vi "Passive Force Clamp-final-v1.vi"(4 "file name add to the end (height)":string="h300", 5 "feedback?":bool, 6 "X=T,Y=F":bool=TRUE, 7 "save?":bool, 8 "Intensity Control, 0~-7000 (mV)":dbl=-1200.0 format="%_8g", 9 "moving step size (um)":dbl=0.05, 10 "upper set value":dbl=0.34, 11 "range (um)":dbl=2.0 format="%.3f") -> ()   [LabVIEW 2014]
uses:
  <vilib>/Analysis/baseanly.llb/Mean (DBL).vi
  Main-Stage-PI/(Global) Current handle and LaserPower_YCC.vi
  <vilib>/Analysis/NI_AALBase.lvlib
panel:
  in  "Custom choose?":bool
  out "Jump to middle (um)":dbl
  out "Max QPD-Stage Pos (um)":dbl
  in  "lower set value":dbl=0.26
  out "target QPD (V)":dbl
  in  "Avg. time delay (ms)":dbl=20.0
  out "True Target position":dbl
  in  "averged delay":dbl
  out "Record scan rate  (um/s)":dbl=2.0
  out "Laser Lock?":bool
  out "Center QPD yc (V)":dbl format="%0.2f"
  out "Sampling rate after filtering (Hz)":dbl
  in  "Who's Data":enum16{"YCC", "PYW", "LCH", "YYH"}(ring)
  in  "left rank":i32=160
  out "Stage-QPD data":dbl[][](array[numeric])
  out "Now position (um)":dbl
  in  "Avg points":i32=320
  out "True rate?":bool
  out "Real initial position (um)":dbl format="%0.5f"
  out "Axis":i32
  in  "toward+ ?\nT=+, F=-":bool
  out "target position (um)":dbl
  in  "stop":bool
  in  "Tab Control":enum32{"Stage movment", "Raw Data", "All Data"}(tab)
  out "XY Graph":T1(graph)
  in  "Set Target position?":bool
  out "Z-QPD":dbl(graph)
  out "Waveform Chart":dbl[](graph)
  out "XY Graph 2":cluster{dbl[], "Filtered X":dbl[]}[](graph)
  in  "Sampling rate":dbl=32000.0
  # "20R-- 300mV"
  # "peak~350 nm\nfrom r = 400 to 500 nm"
  # "jump to r=450 nm"
  # "2.9um for had acted"
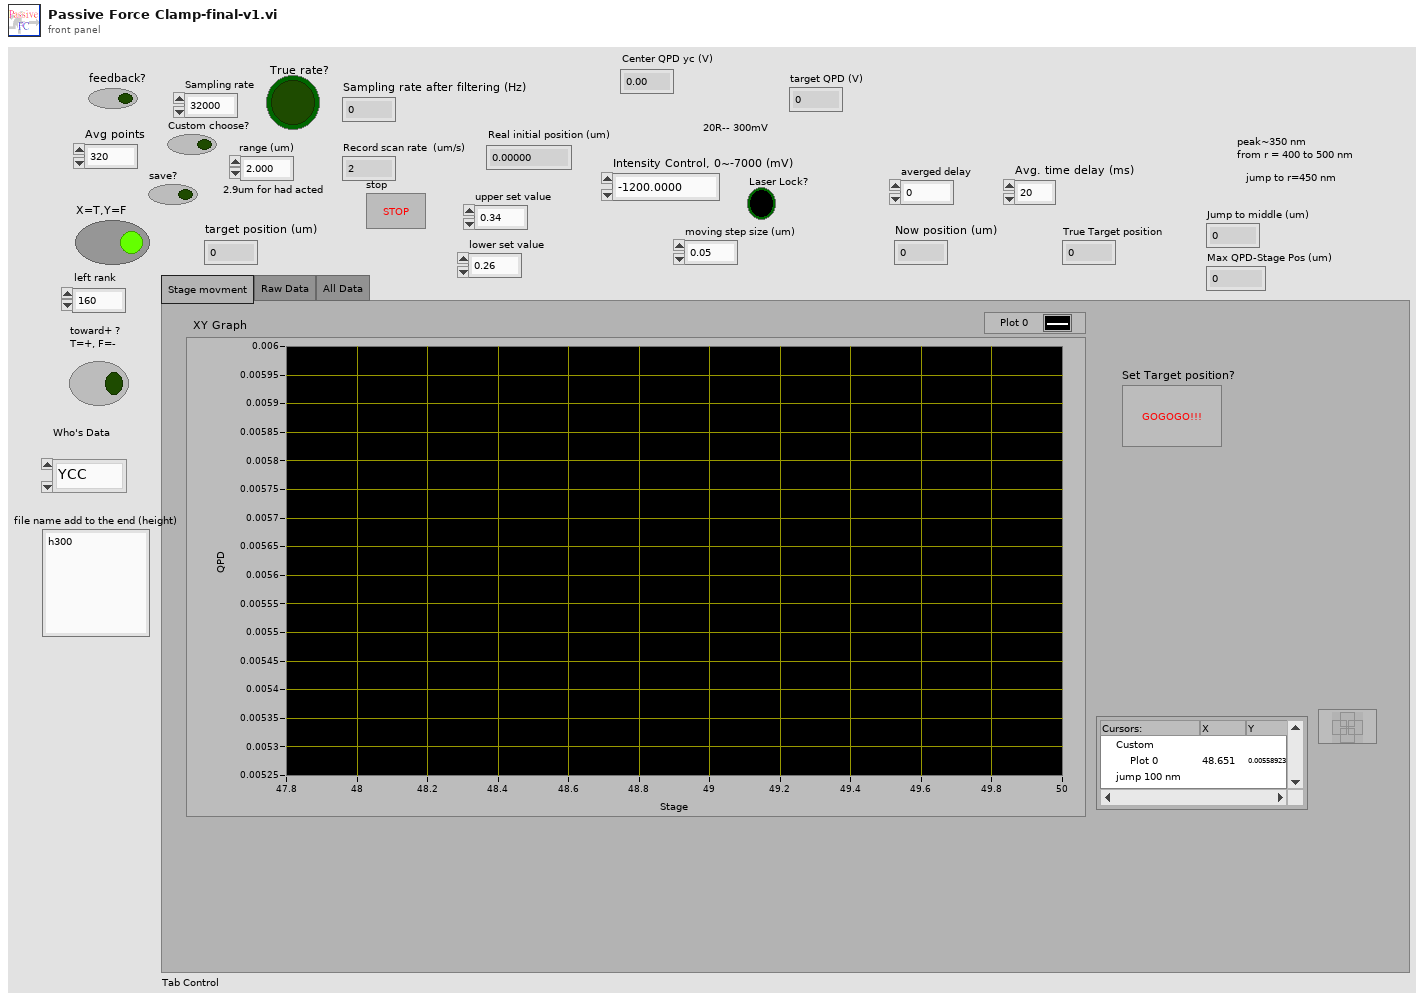
[diagram p1: front panel]
types:
  T1 = cluster{"Filtered Stage Array":dbl[], "Filtered QPD data":dbl[]}
  T2 = enum16{"Fixed-window avg", "Moving-window avg", "F+S-window avg", "S-G filter", "Fixed-window Median", "Moving-window Median "}
  T3 = cluster{"Correct Unfolded Stage Array (um)":dbl[], "Filtered QPD Array":dbl[]}
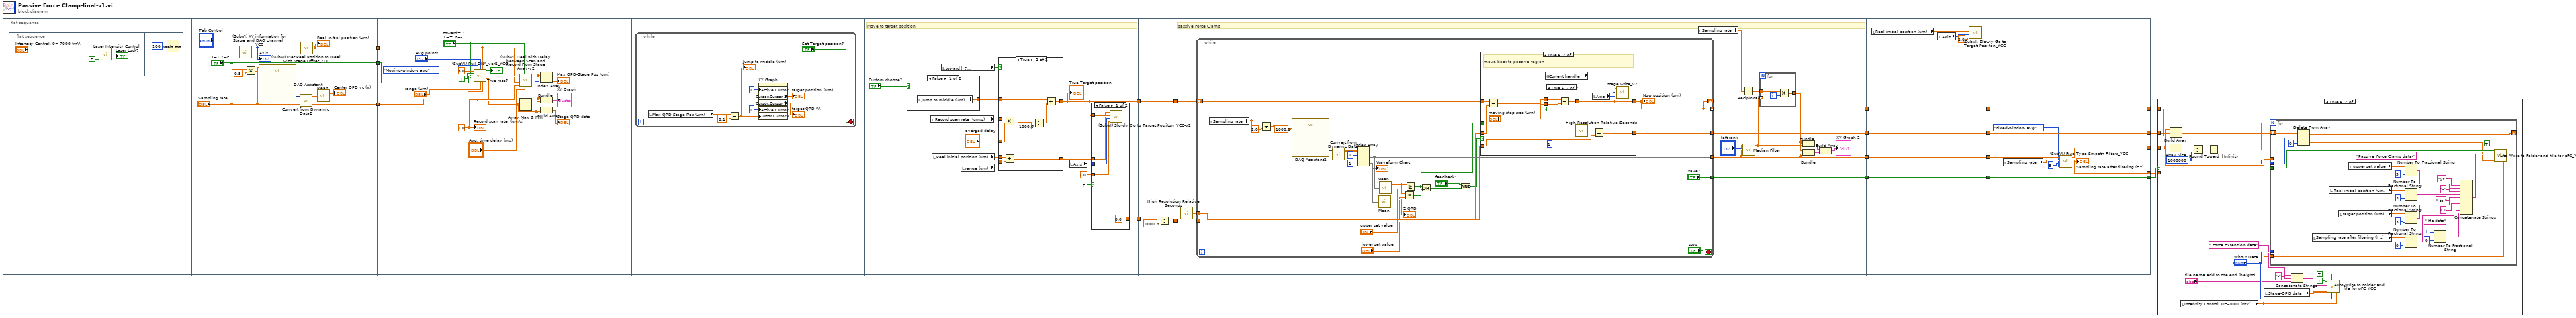
[diagram p0: block diagram]
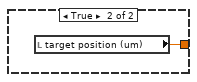
[diagram p3: hidden frame]
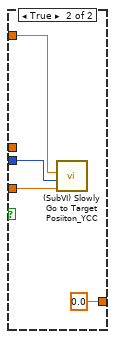
[diagram p4: hidden frame]
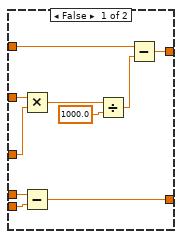
[diagram p5: hidden frame]
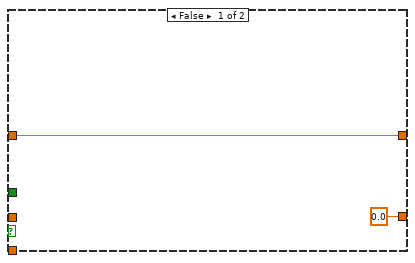
[diagram p6: hidden frame]
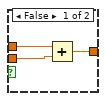
[diagram p7: hidden frame]
diagram:
  n1 = flat-sequence {
    tunnel: [w32] -> w17
    tunnel: ["X=T,Y=F"] -> w16
    tunnel: ["Sampling rate"] -> w5
    tunnel: w17 -> [w40]
    tunnel: w16 -> [w45]
    tunnel: w5 -> [w44]
    tunnel: [w68] -> w15
    tunnel: [w73] -> w4
    tunnel: w15 -> [w108]
    tunnel: [w108] -> w14
    tunnel: [w106] -> w13
    tunnel: w4 -> [w105]
    tunnel: w14 -> [w120]
    tunnel: w13 -> [w119]
    tunnel: [w113] -> w11
    tunnel: [w122] -> w9
    tunnel: [w121] -> w7
    tunnel: [w109] -> w2
    tunnel: w11 -> [w178]
    tunnel: [w178] -> w10
    tunnel: w9 -> [w177]
    tunnel: [w177] -> w8
    tunnel: w7 -> [w176]
    tunnel: [w176] -> w6
    tunnel: [w172] -> w3
    tunnel: w2 -> [w172]
    tunnel: [w186] -> w18
    tunnel: [w187] -> w19
    tunnel: [w181] -> w20
    tunnel: w10 -> [w185]
    tunnel: w8 -> [w187]
    tunnel: w6 -> [w186]
    tunnel: [w182] -> w12
    tunnel: w3 -> [w179]
    tunnel: [w179] -> w1
    frame #0 {
      n2 = flat-sequence {
        frame #0 {
          n3 = call "Laser Intensity Control.vi"("Close?"=FALSE, "Intensity Control, 0~-7000 (mV)"="Intensity Control, 0~-7000 (mV)") -> ("Laser Lock?"=→"Laser Lock?":bool)  [unwired: 5 in]
        }
        frame #1 {
          n4 = Wait (ms)(milliseconds to wait=u32 100) -> ()  [unwired: 1 out]
        }
      }
    }
    frame #1 {
      n5 = call "(SubVI) XY information for Stage and DAQ channel_YCC.vi"("T=X\nF=Y"="X=T,Y=F") -> ("Axis"=w33:i32)  [unwired: 3 in, 1 out]
      "Axis" <- w33
      n6 = Multiply(x="Sampling rate", y=0.5) -> (x*y=w28:dbl)
      n7 = call "DAQ Assistant"("rate"="Sampling rate", "number of samples"=w28) -> ("data"=w27:dynamicdata)  [unwired: 15 in, 2 out]
      n8 = call "Convert from Dynamic Data2"("Dynamic Data Type"=w27) -> ("Array"=w26:dbl[])  [unwired: 3 in]
      n9 = call "(SubVI) Get Real Position to Deal with Stage Offset_YCC.vi"("Axis"=w33) -> ("Real Current Commanded position (um)"=w32:dbl)  [unwired: 3 in, 1 out]
      "Real initial position (um)" <- w32
      n10 = call-poly <vilib>:"Mean.vi"("X"=w26) -> ("mean"=→"Center QPD yc (V)":dbl)  [unwired: 1 out]
    }
    frame #2 {
      w39 = 1.0 ("Record scan rate  (um/s)")
      n11 = call "(SubVI) Pull DNA_ver2_YCC.vi"("waiting time per point (ms)\nrange from 5ms to 0.167 ms"=5.0 ("waiting time per point (ms)\nrange from 5ms to 0.167 ms"), "Filter type"=T2."Moving-window avg", "Avg points"="Avg points", "Real initial position (um)"=w40, "Record?"=TRUE, "T=X\nF=Y"=w45, "Toward  ?\nT=+, F=-"="toward+ ?\nT=+, F=-", "Record scan rate  (um/s)"=w39, "range  (um)"="range (um)", "Sampling rate"=w44) -> ("True rate?"=→"True rate?":bool, "Filtered Stage Array"=w42:dbl[], "Filtered QPD Array"=w37:dbl[])  [unwired: 2 in, 1 out]
      n12 = call "(SubVI) Deal with Delay between Scan and Record From Stage Array-v2.vi"("Avg. time delay (ms)"="Avg. time delay (ms)", "Toward first ?\nT=+, F=-"="toward+ ?\nT=+, F=-", "Record scan rate  (um/s)"=w39, "Real initial position (um)"=w40, "Unfolded Stage Array (um)"=w42) -> ("Correct Unfolded Stage Array (um)"=w36:dbl[])  [unwired: 2 in, 2 out]
      n13 = Array Max & Min(array=w37) -> (max index (indices)=w35:i32)  [unwired: 3 out]
      n14 = Index Array(array=w36, index=w35) -> (element=→"Max QPD-Stage Pos (um)":dbl)
      n15 = Bundle("Correct Unfolded Stage Array (um)"=w36, "Filtered QPD Array"=w37) -> (→"XY Graph":T3)  [unwired: 1 in]
      n16 = Build Array(w36, w37) -> (→"Stage-QPD data":dbl[][])
      "Record scan rate  (um/s)" <- w39
    }
    frame #3 {
      n17 = while {
        stop <- "Set Target position?" stop-if-true
        n18 = local read "Max QPD-Stage Pos (um)"() -> (w55:dbl)
        n19 = Subtract(x=w55, y=0.1) -> (x-y=w53:dbl)
        "Jump to middle (um)" <- w53
        n20 = property on="XY Graph" class="XYGraph (strict)"("Active Cursor"=u32 0, "Active Cursor"=u32 1, "Cursor.Cursor X"=w53) -> ("Cursor.Cursor X"=→"target position (um)":dbl, "Cursor.Cursor Y"=→"target QPD (V)":dbl)  [unwired: 2 in, 2 out]
      }
    }
    frame #4 {
      # "Move to target position"
      n21 = case shown="False" "Custom choose?" {
        tunnel: [w74 w75] -> w72
        frame False {
          n22 = local read "Jump to middle (um)"() -> (w74:dbl)
        }
        frame True {
          n23 = local read "target position (um)"() -> (w75:dbl)
        }
      }
      n24 = local read "Record scan rate  (um/s)"() -> (w69:dbl)
      n25 = local read "Real initial position (um)"() -> (w64:dbl)
      n26 = local read "toward+ ?\nT=+, F=-"() -> (w71:bool)
      n27 = local read "range (um)"() -> (w63:dbl)
      n28 = case shown="True" w71 {
        tunnel: w72 -> [w94 w100]
        tunnel: [w90 w98] -> w68
        tunnel: "averged delay" -> [w89 w101]
        tunnel: w69 -> [w88 w102]
        tunnel: w64 -> [w87 w97]
        tunnel: w63 -> [w86 w96]
        tunnel: [w85 w95] -> w62
        frame False {
          n29 = Multiply(x=w88, y=w89) -> (x*y=w93:dbl)
          n30 = Subtract(x=w87, y=w86) -> (x-y=w85:dbl)
          n31 = Divide(x=w93, y=1000.0) -> (x/y=w91:dbl)
          n32 = Subtract(x=w94, y=w91) -> (x-y=w90:dbl)
        }
        frame True {
          n33 = Multiply(x=w102, y=w101) -> (x*y=w104:dbl)
          n34 = Add(x=w97, y=w96) -> (x+y=w95:dbl)
          n35 = Divide(x=w104, y=1000.0) -> (x/y=w99:dbl)
          n36 = Add(x=w100, y=w99) -> (x+y=w98:dbl)
        }
      }
      "True Target position" <- w68
      n37 = local read "Axis"() -> (w66:i32)
      n38 = case shown="False" FALSE {
        tunnel: [0.0 ("Expect - Real move (nm)\nStage Offset\n+=more move\n-=less move") 0.0 ("Expect - Real move (nm)\nStage Offset\n+=more move\n-=less move")] -> w73
        tunnel: w68 -> [w79 w84]
        tunnel: w66 -> [w78 w82]
        tunnel: 1.0 ("scan rate  (um/s)") -> [w77 w81]
        tunnel: w62 -> [w76 _]
        frame False {
          n39 = call "(SubVI) Slowly Go to Target Posiiton_YCC-v2.vi"("scan rate  (um/s)"=w77, "axis"=w78, "Target position (um)"=w79, "Now position (um)"=w76) -> ()  [unwired: 2 in, 2 out]
        }
        frame True {
          n40 = call "(SubVI) Slowly Go to Target Posiiton_YCC.vi"("scan rate  (um/s)"=w81, "axis"=w82, "Target position (um)"=w84) -> ()  [unwired: 1 in, 4 out]
        }
      }
    }
    frame #5 {
      n41 = Divide(x=w105, y=1000.0) -> (x/y=w106:dbl)
    }
    frame #6 {
      # "passive Force Clamp"
      n42 = call <vilib>:"High Resolution Relative Seconds.vi"() -> ("relative seconds"=w123:dbl)
      n43 = while {
        tunnel: w123 -> [w149]
        tunnel: [w148] -> w122 mode=indexing
        tunnel: [w135] -> w113 mode=concatenating
        tunnel: ["save?"] -> w121
        shift-right: [w127] -> _
        shift-left: w120 -> [w139]
        tunnel: w119 -> [w140]
        tunnel: [w127] -> w109 mode=indexing
        stop <- "stop" stop-if-true
        n44 = local read "Sampling rate"() -> (w143:dbl)
        n45 = Divide(x=w143, y=2.0) -> (x/y=w141:dbl)
        n46 = call "DAQ Assistant2"("rate"=w143, "number of samples"=w141, "timeout (s)"=1000.0) -> ("data"=w146:dynamicdata)  [unwired: 13 in, 3 out]
        n47 = call "Convert from Dynamic Data"("Dynamic Data Type"=w146) -> ("Array"=w138:dbl[][])  [unwired: 3 in]
        n48 = Index Array(array=w138, index (row) #1=0 ("index (row)"), index (row) #2=1 ("index (row)")) -> (element #1=w135:dbl[], element #2=w134:dbl[])  [unwired: 2 in]
        "Waveform Chart" <- w135
        n49 = call-poly <vilib>:"Mean.vi"("X"=w134) -> ("mean"=→"Z-QPD":dbl)  [unwired: 1 out]
        n50 = call-poly <vilib>:"Mean.vi"("X"=w135) -> ("mean"=w151:dbl)  [unwired: 1 out]
        n51 = Less Or Equal?(x=w151, y="lower set value") -> (x <= y?=w130:bool)
        n52 = Greater Or Equal?(x=w151, y="upper set value") -> (x >= y?=w128:bool)
        n53 = Or(x=w128, y=w130) -> (x .or. y?=w129:bool)
        n54 = And(x="feedback?", y=w129) -> (x .and. y?=w131:bool)
        n55 = case shown="True" w131 {
          tunnel: w149 -> [_ w164]
          tunnel: [0.0 w162] -> w148
          tunnel: [w153 w161] -> w127
          tunnel: w140 -> [_ w159]
          tunnel: w139 -> [w153 w156]
          tunnel: w128 -> [_ w155]
          frame False {
          }
          frame True {
            (unwired) 1 ("read #")
            # "move back to passive region"
            n56 = Subtract(x=w156, y=w159) -> (x-y=w158:dbl)
            n57 = case shown="True" w155 {
              tunnel: "moving step size (um)" -> [w166 w171]
              tunnel: [w168 w170] -> w161
              tunnel: w158 -> [w167 w169]
              frame False {
                n58 = Add(x=w167, y=w166) -> (x+y=w168:dbl)
              }
              frame True {
                n59 = Subtract(x=w169, y=w171) -> (x-y=w170:dbl)
              }
            }
            n60 = global read "(Global) Current handle and LaserPower_YCC.vi" "Current handle"() -> (w157:i32)
            n61 = call <vilib>:"High Resolution Relative Seconds.vi"() -> ("relative seconds"=w163:dbl)
            n62 = local read "Axis"() -> (w160:i32)
            n63 = Subtract(x=w163, y=w164) -> (x-y=w162:dbl)
            n64 = call "stage write_v2.vi"("axis"=w160, "Incoming Handle"=w157, "position"=w161) -> ()  [unwired: 2 in, 1 out]
          }
        }
        "Now position (um)" <- w127
      }
      n65 = local read "Sampling rate"() -> (w117:dbl)
      n66 = Reciprocal(x=w117) -> (1/x=w116:dbl)
      n67 = call <vilib>:"Median Filter.vi"("left rank"="left rank", "X"=w113) -> ("Filtered X"=w115:dbl[])  [unwired: 8 in, 1 out]
      n68 = for {
        tunnel: w115 -> [_] mode=indexing
        tunnel: w116 -> [w125]
        tunnel: [w124] -> w114 mode=indexing
        i -> [w126]
        n69 = Multiply(x=w125, y=w126) -> (x*y=w124:dbl)
      }
      n70 = Bundle(w114, "Filtered X"=w115) -> (w111:cluster{dbl[], "Filtered X":dbl[]})  [unwired: 1 in]
      n71 = Bundle(w114, "Array"=w113) -> (w110:cluster{dbl[], "Array":dbl[]})  [unwired: 1 in]
      n72 = Build Array(w111, w110) -> (→"XY Graph 2":cluster{dbl[], "Array":dbl[]}[])
    }
    frame #7 {
      n73 = local read "Real initial position (um)"() -> (w174:dbl)
      n74 = local read "Axis"() -> (w175:i32)
      n75 = call "(SubVI) Slowly Go to Target Posiiton_YCC.vi"("scan rate  (um/s)"=2.0, "axis"=w175, "Target position (um)"=w174) -> ()  [unwired: 1 in, 4 out]
    }
    frame #8 {
      n76 = local read "Sampling rate"() -> (w184:dbl)
      n77 = call "(SubVI) Five-Type Smooth Filters_YCC.vi"("Filter type"=T2."Fixed-window avg", "Avg points"=8, "Sampling rate (Hz)"=w184, "QPD data"=w185) -> ("Sampling rate after filtering (Hz)"=w182:dbl, "Filtered QPD data"=w181:dbl[])  [unwired: 1 in]
      "Sampling rate after filtering (Hz)" <- w182
    }
  }
  n78 = case shown="True" w18 {
    selector: w18 -> [_ w205]
    tunnel: w20 -> [_ w201]
    tunnel: w19 -> [_ w200]
    tunnel: w12 -> [_ _]
    tunnel: w1 -> [_ w188]
    frame False {
    }
    frame True {
      w198 = 1000000 ("y")
      n79 = Build Array(w201, w200, w188) -> (w199:dbl[][])
      n80 = Array Size(array=w201) -> (size(s)=w202:i32)
      n81 = local read "Intensity Control, 0~-7000 (mV)"() -> (w189:dbl)
      n82 = Divide(x=w202, y=w198) -> (x/y=w204:dbl)
      n83 = Round Toward +Infinity(x=w204) -> (ceil(x): smallest int >= x=w203:dbl)
      n84 = local read "Stage-QPD data"() -> (w197:dbl[][])
      n85 = for {
        N: w203 -> [_]
        tunnel: w201 -> [_]
        tunnel: w205 -> [w227]
        shift-right: [w213] -> _
        shift-left: w199 -> [w218]
        tunnel: w198 -> [w217]
        tunnel: "Who's Data" -> [w212]
        tunnel: w189 -> [w206]
        i -> [w225]
        n86 = Delete From Array(array=w218, length=w217, index (col)=0 ("index (row)")) -> (deleted portion=w215:dbl[][], array with subset deleted=w213:dbl[][])  [unwired: 1 in]
        n87 = local read "Sampling rate after filtering (Hz)"() -> (w226:dbl)
        n88 = local read "Real initial position (um)"() -> (w236:dbl)
        n89 = local read "target position (um)"() -> (w233:dbl)
        n90 = local read "upper set value"() -> (w209:dbl)
        n91 = Number To Fractional String(number=w209, precision (6)=i16 5) -> (F-format string=w207:string)  [unwired: 2 in]
        n92 = Number To Fractional String(number=w236, precision (6)=i16 3) -> (F-format string=w232:string)  [unwired: 2 in]
        n93 = Number To Fractional String(number=w233, precision (6)=i16 3) -> (F-format string=w230:string)  [unwired: 2 in]
        n94 = Number To Fractional String(number=w226, precision (6)=i16 0) -> (F-format string=w221:string)  [unwired: 2 in]
        n95 = Number To Fractional String(number=w225, precision (6)=i16 0) -> (F-format string=w219:string)  [unwired: 2 in]
        n96 = Concatenate Strings("Passive Force Clamp data-" ("prompt"), "yt " ("string"), w207, "-" ("string"), w232, " to " ("string"), w230, "-" ("string"), w221, " Hz-data" ("string"), w219) -> (w228:string)
        n97 = call "Auto-Write to Folder and file for pFC_YCC.vi"("Current PD (mV)"=w206, "Who's Data"=w212, "T=2D\nF=1D"=TRUE ("T=2D\nF=1D"), "2D data to be saved"=w215, "File name add to the end \n(height)"=w228, "Save?"=w227) -> ()  [unwired: 2 in, 2 out]
      }
      n98 = Concatenate Strings(" Force Extension data" ("prompt"), "-" ("string"), "file name add to the end (height)") -> (w190:string)
      n99 = call "Auto-Write to Folder and file for pFC_YCC.vi"("Current PD (mV)"=w189, "Who's Data"="Who's Data", "T=2D\nF=1D"=TRUE ("T=2D\nF=1D"), "2D data to be saved"=w197, "File name add to the end \n(height)"=w190, "Save?"=TRUE) -> ()  [unwired: 2 in, 2 out]
    }
  }
